vi "ErrorHandling.Fglb.Get.vi"(8 "error in (no error)":errorcluster) -> (0 "error out":errorcluster, 2 "Errors":T1[](array[typedef]), 3 "unconfirmed?":bool)   [LabVIEW 2016]
uses:
  CitTemplate/citTemplate.errData.ctl
  EventLog/EventLog.EventSource.ctl
  ErrorHandling.Fglb.Action.ctl
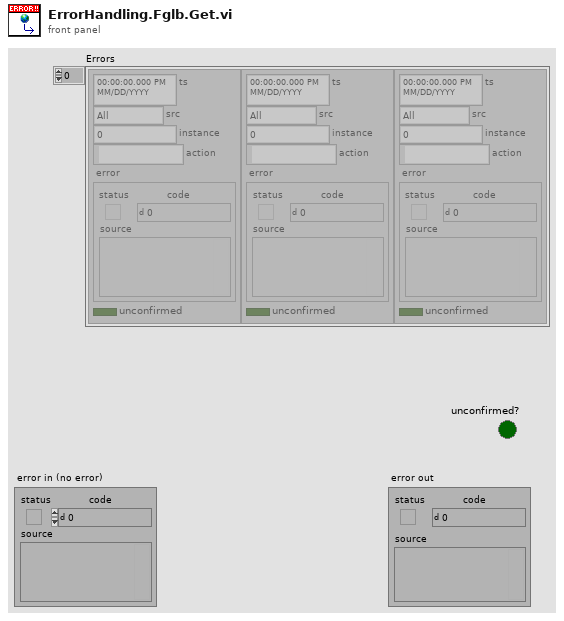
[diagram p1: front panel]
types:
  T1 = typedef "citTemplate.errData.ctl" = cluster{"ts":timestamp, "src":T2, "instance":i32, "action":string, "error":errorcluster, "unconfirmed":bool}
  T2 = typedef "EventLog.EventSource.ctl" = enum16{"All", "Gui", "Cache", "PLC1", "PLC2", "PLC3", "DB", "DB01", "DB02", "DB03", "DB04", "DB05", "DB06", "DB07", "DB08", "DB09", "DB10", "DB11", "DB12", "DB13", "DB14", "DB15", "DB16"}
  T3 = typedef "ErrorHandling.Fglb.Action.ctl" = enum16{"init", "add", "clear", "confirm", "check", "get"}
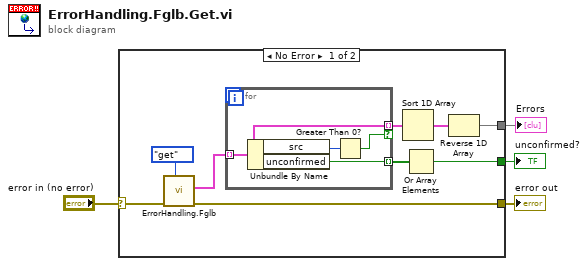
[diagram p0: block diagram]
diagram:
  n1 = case shown="No Error" "error in (no error)" {
    selector: "error in (no error)" -> [w11 w18]
    tunnel: [w12 w18] -> w4
    tunnel: [w5 _] -> w2
    tunnel: [w7 _] -> w1
    frame No Error {
      n2 = call "ErrorHandling.Fglb.vi"("Action"=ErrorHandling.Fglb.Action."get", "error in (no error)"=w11) -> ("error out"=w12:errorcluster, "Errors out"=w9:T1[])  [unwired: 7 in, 1 out]
      n3 = for {
        tunnel: w9 -> [w17] mode=indexing
        tunnel: [w17] -> w10 mode=indexing if=w15
        tunnel: [w14] -> w8 mode=indexing
        n4 = Unbundle By Name(w17) -> ("src"=w16:T2, "unconfirmed"=w14:bool)
        n5 = Greater Than 0?(x=w16) -> (x > 0?=w15:bool)
      }
      n6 = Sort 1D Array(array=w10) -> (sorted array=w6:T1[])
      n7 = Or Array Elements(Boolean array=w8) -> (logical OR=w7:bool)
      n8 = Reverse 1D Array(array=w6) -> (reversed array=w5:T1[])
    }
    frame Error {
    }
  }
  "error out" <- w4
  "Errors" <- w2
  "unconfirmed?" <- w1
